vi "readFromXML.vi"(8 "error in (no error)":errorcluster, 10 "XMLin":string, 11 "GuideClear in":refnum<class "GuideClear.lvclass">) -> (0 "error out":errorcluster, 3 "GuideClear out":refnum<class "GuideClear.lvclass">)   [LabVIEW 2014, in "TCSDataDefinitions.lvlib" / "TCSCommand.lvlib" / "GuiderCommands.lvlib" / "GuideClear.lvclass"]
uses:
  GuideClear.lvclass
  GuiderCommands.lvclass
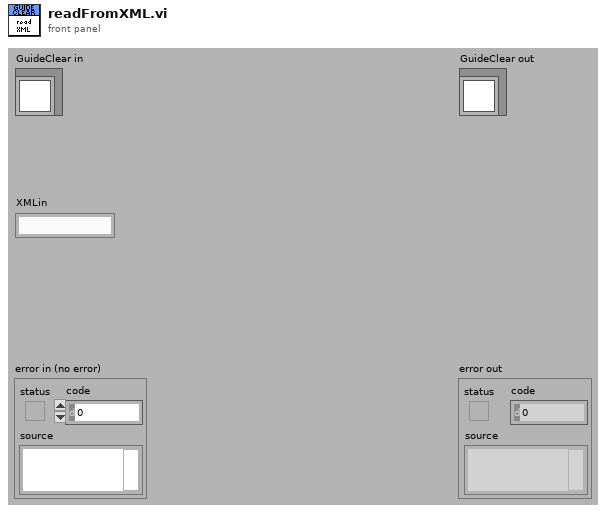
[diagram p1: front panel]
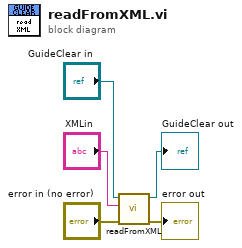
[diagram p0: block diagram]
diagram:
  n1 = call-parent "readFromXML.vi"("error in (no error)"="error in (no error)", "XMLin"="XMLin", "GuiderCommands in"="GuideClear in") -> ("error out"=→"error out":errorcluster, "GuiderCommands out"=→"GuideClear out":refnum<class "GuideClear.lvclass">)  [unwired: 7 in]
